vi "fromString.vi"(9 "DateTime String":string, 11 "DateTime.ISO8601 in":refnum<class "DateTime.ISO8601.lvclass">) -> (1 "Timestamp":timestamp, 3 "DateTime.ISO8601 out":refnum<class "DateTime.ISO8601.lvclass">)   [LabVIEW 2018, in "DateTime.ISO8601.lvclass"]
uses:
  DateTime.ISO8601.lvclass
  DateTime.ISO8601.lvclass/DateTime.ISO8601.ctl
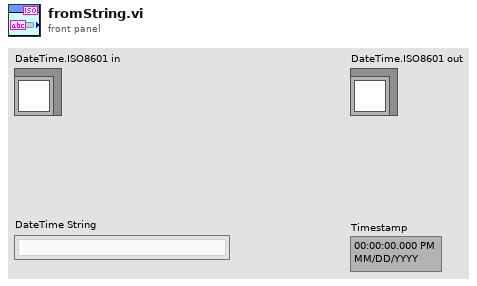
[diagram p1: front panel]
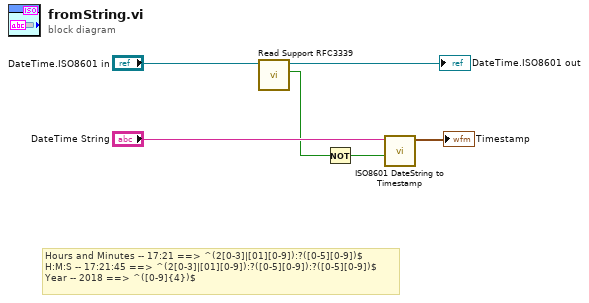
[diagram p0: block diagram]
diagram:
  # "Hours and Minutes -- 17:21 ==> ^(2[0-3]|[01][0-9]):?([0-5][0-9])$\nH:M:S -- 17:21:45 ==> ^(2[0-3]|[01][0-9]):?([0-5][0-9]):?([0-5][0-9])$\nYear -- 2018 ==> ^([0-9]{4})$"
  n1 = call "Read Support RFC3339.vi"("DateTime.ISO8601 in"="DateTime.ISO8601 in") -> ("Support RFC3339"=w3:bool, "DateTime.ISO8601 out"=→"DateTime.ISO8601 out":refnum<class "DateTime.ISO8601.lvclass">)  [unwired: 9 in]
  n2 = Not(x=w3) -> (.not. x?=w2:bool)
  n3 = call "ISO8601 DateString to Timestamp.vi"("Strict ISO? (T)"=w2, "ISO8601 Date String"="DateTime String") -> ("Timestamp"=→"Timestamp":timestamp)  [unwired: 7 in, 2 out]
